vi "Post Steptypes Power Monitor Stop.vi"(11 "Sequence Context In":refnum<k7>) -> (0 "error out":errorcluster, 3 "Report Text":string)   [LabVIEW 2023, in "LTT_TeststandSteptypes.lvlib"]
uses:
  LTT_TeststandSteptypes.lvlib
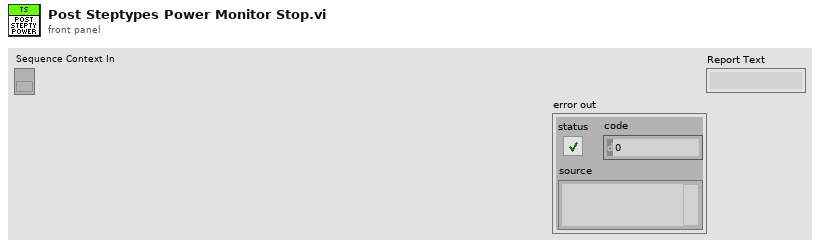
[diagram p1: front panel]
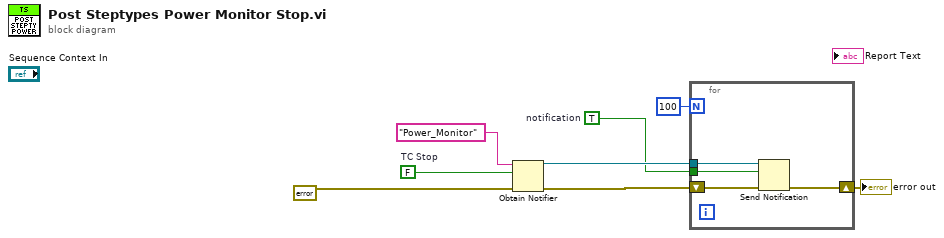
[diagram p0: block diagram]
diagram:
  w3 = TRUE  # notification
  w7 = FALSE  # TC Stop
  n1 = Obtain Notifier(name (unnamed)="Power_Monitor", notification data type=w7, error in (no error)=errorcluster {"status"=FALSE, "code"=0, "source"=""}) -> (notifier out=w5:refnum<notifier>, error out=w4:errorcluster)  [unwired: 1 in, 1 out]
  n2 = for {
    N: 100 -> [_]
    tunnel: w5 -> [w12]
    tunnel: w3 -> [w10]
    shift-right: [w9] -> w2
    shift-left: w4 -> [w11]
    n3 = Send Notification(notification=w10, notifier=w12, error in (no error)=w11) -> (error out=w9:errorcluster)  [unwired: 1 out]
  }
  "error out" <- w2
